vi "Construct Listbox Item Names Binding.vi"(9 "Set to top upon write? (F)":T1, 10 "LstBox Refnum":refnum<vi>) -> (0 "error out":errorcluster, 3 "ListboxItemNamesBinding":refnum<class "ListboxItemNamesBinding.lvclass">)   [LabVIEW 2017, in "ListboxItemNamesBinding.lvclass"]
doc: "<License>\nCopyright © 2017 Composed Systems, LLC | All rights reserved\nwww.composed.io\n\nAuthor: Ethan Stern <ethan.stern@composed.io>\n\nThis software is provided \"AS IS\" WITHOUT WARRANTIES, either express or implied, AND IS FOR EDUCATIONAL PURPOSES ONLY.\n</License>"
uses:
  ListboxItemNamesBinding.lvclass
  Listbox Binding Options.ctl
  ListboxItemNamesBinding.lvclass/ListboxItemNamesBinding.ctl
  <vilib>/Utility/error.llb/Error Cluster From Error Code.vi
  <vilib>/ErrorRing/Error Ring.xnode
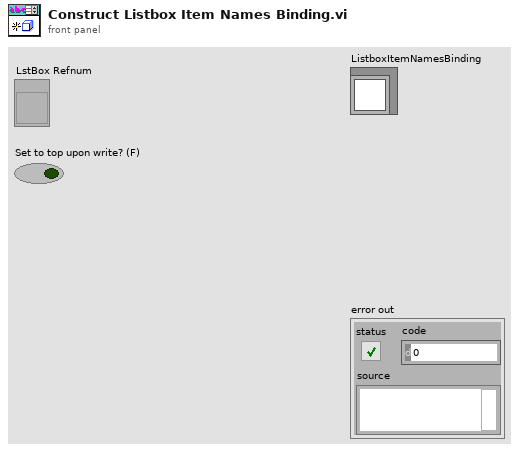
[diagram p1: front panel]
types:
  T1 = typedef "ListboxItemNamesBinding.lvclass/Listbox Binding Options.ctl" = bool
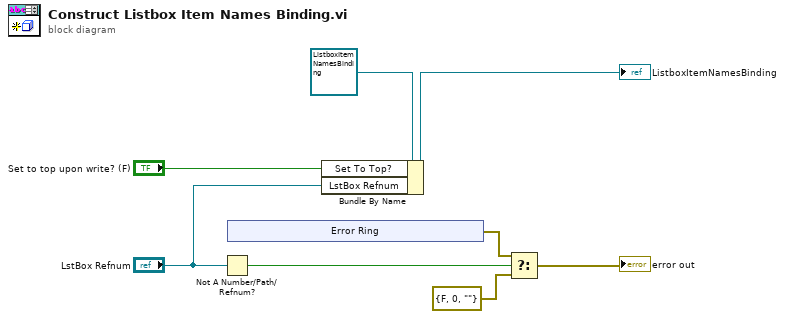
[diagram p0: block diagram]
diagram:
  n1 = Not A Number/Path/Refnum?(number/path/refnum="LstBox Refnum") -> (NaN/Path/Refnum?=w4:bool)
  n2 = xnode "Error Ring"() -> ("error out"=w1:errorcluster)
  n3 = Bundle By Name(cluster=refnum<class "ListboxItemNamesBinding.lvclass"> refnum ("ListboxItemNamesBinding"), "Set To Top?"="Set to top upon write? (F)", "LstBox Refnum"="LstBox Refnum") -> (→"ListboxItemNamesBinding":refnum<class "ListboxItemNamesBinding.lvclass">)
  n4 = Select(t=w1, s=w4, f=errorcluster {"status"=FALSE, "code"=0, "source"=""} ("error constant")) -> (s? t:f=→"error out":errorcluster)
